vi "dotNetExceptionStringWrapper.vi"(0 "ExceptionIn":string="Error calling method Konvolucio.MCAN120803.MCanAdapter.ConnectTo, (System.Reflection.TargetInvocationException: A meghívott objektum kivételt váltott ki.\n\tInner Exception: Konvolucio.MCAN120803.MCanAdapterException: Adapter not found by Serial Number. Code:-8603.) <append><b>Konvolucio.MCAN120803.MCanAdapterException</b> in Konvolucio MCAN120803.lvlib:ConnectBySerialNumber.vi->Konvolucio MCAN120803 Example_0003 ConnectBySerialNumber.vi") -> (2 "Code":i32, 3 "ExceptionOut":string)   [LabVIEW 2011, in "Konvolucio MCAN120803.lvlib"]
uses:
  <instrlib>/Konvolucio MCAN120803/Konvolucio MCAN120803.lvlib
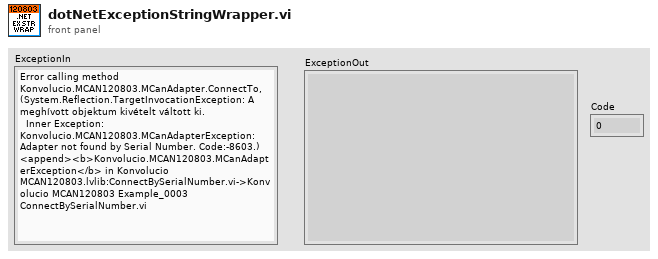
[diagram p1: front panel]
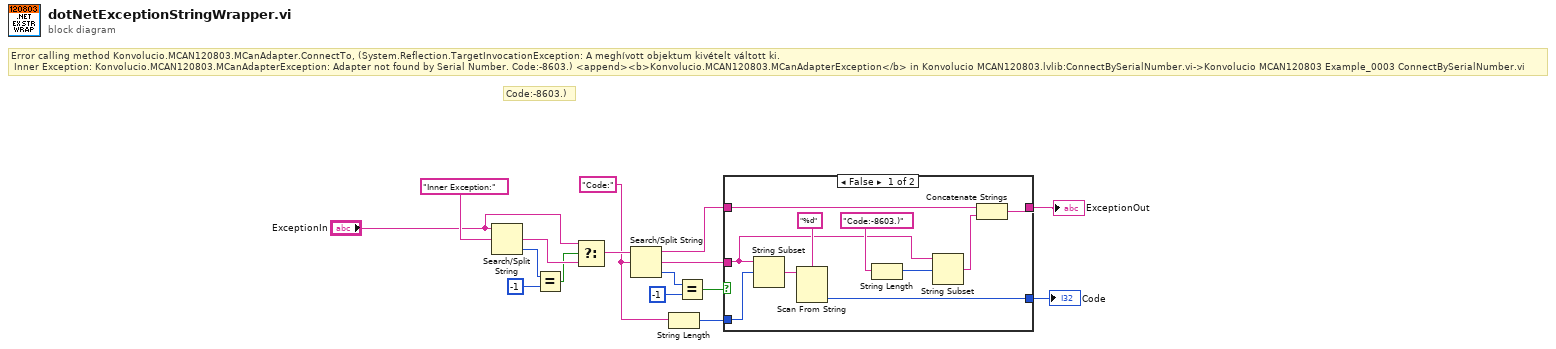
[diagram p0: block diagram]
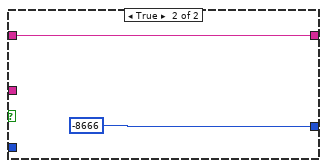
[diagram p2: hidden frame]
diagram:
  w5 = "Code:" ("search string/char (-)")
  # "Code:-8603.)"
  # "Error calling method Konvolucio.MCAN120803.MCanAdapter.ConnectTo, (System.Reflection.TargetInvocationException: A meghívott objektum kivételt váltott ki.\n\tInner Exception: Konvolucio.MCAN120803.MCanAdapterException: Adapter not found by Serial Number. Code:-8603.) <append><b>Konvolucio.MCAN120803.MCanAdapterException</b> in Konvolucio MCAN120803.lvlib:ConnectBySerialNumber.vi->Konvolucio MCAN120803 Example_0003 ConnectBySerialNumber.vi"
  n1 = Search/Split String(string="ExceptionIn", search string/char (-)="Inner Exception:") -> (match + rest of string=w16:string, offset of match=w14:i32)  [unwired: 1 in, 1 out]
  n2 = Equal?(x=w14, y=-1) -> (x = y?=w13:bool)
  n3 = Select(t="ExceptionIn", s=w13, f=w16) -> (s? t:f=w10:string)
  n4 = Search/Split String(string=w10, search string/char (-)=w5) -> (substring before match=w2:string, match + rest of string=w6:string, offset of match=w8:i32)  [unwired: 1 in]
  n5 = String Length(string=w5) -> (length=w4:i32)
  n6 = Equal?(x=w8, y=-1) -> (x = y?=w7:bool)
  n7 = case shown="False" w7 {
    tunnel: w6 -> [w20 _]
    tunnel: w4 -> [w26 _]
    tunnel: [w23 -8666 ("y")] -> w3
    tunnel: w2 -> [w19 w27]
    tunnel: [w17 w27] -> w1
    frame False {
      n8 = String Subset(string=w20, offset (0)=w26) -> (substring=w25:string)  [unwired: 1 in]
      n9 = Scan From String(format string="%d", input string=w25) -> (output 1=w23:i32)  [unwired: 3 in, 3 out]
      n10 = String Length(string="Code:-8603.)" ("format string")) -> (length=w21:i32)
      n11 = String Subset(string=w20, offset (0)=w21) -> (substring=w18:string)  [unwired: 1 in]
      n12 = Concatenate Strings(w19, w18) -> (w17:string)
    }
    frame True {
    }
  }
  "Code" <- w3
  "ExceptionOut" <- w1
